vi "Select Excitation Channel.vi"(11 "Sensor List":refnum<class "Sensor List Class.lvclass">) -> (2 "Channel Out":string, 3 "Sensor List Out":refnum<class "Sensor List Class.lvclass">)   [LabVIEW 2013]
uses:
  lib/Data Access Objects/Sensors/Sensor List Class.lvclass
  lib/Data Access Objects/Sensors/Sensor DAO Class.lvclass/Sensor DAO Class.ctl
  <vilib>/regexp/Match Regular Expression.xnode
  lib/Data Access Objects/Sensors/Sensor DAO Class.lvclass
panel:
  in  "Select Excitation Channel":i32[](listbox)
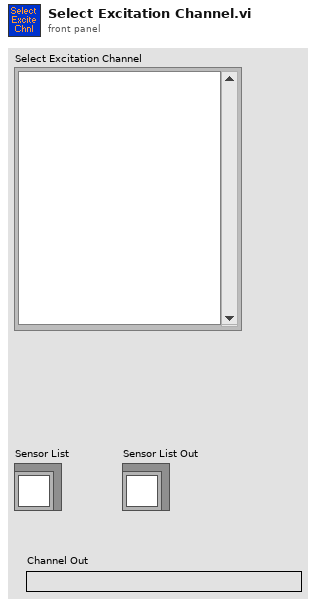
[diagram p1: front panel]
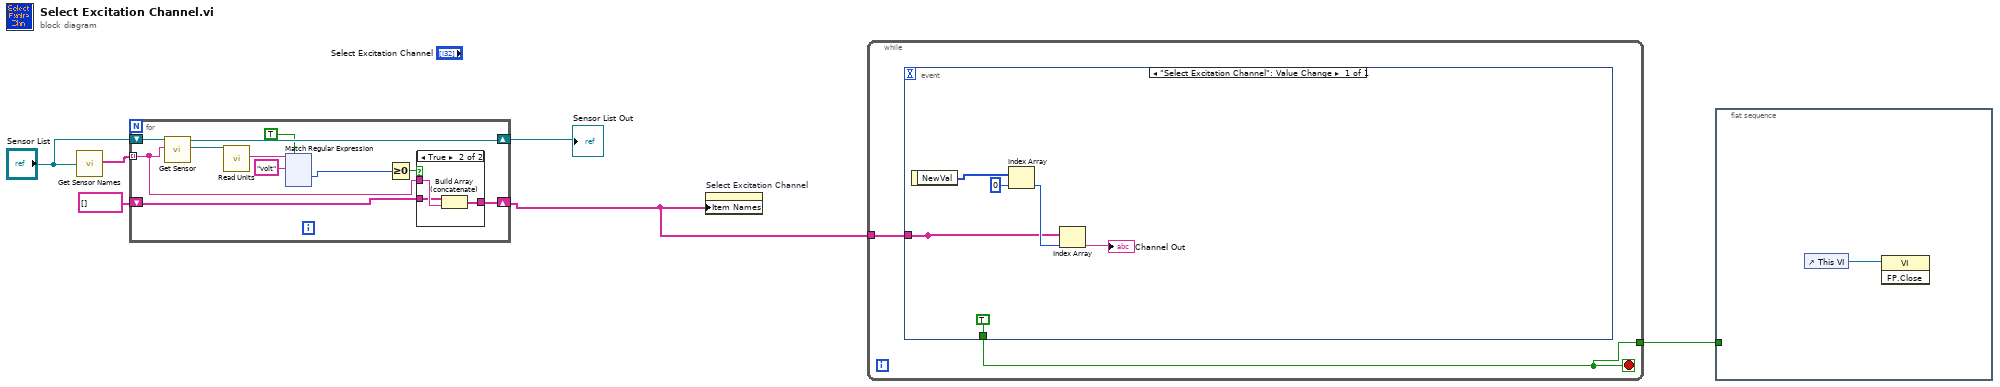
[diagram p0: block diagram]
diagram:
  n1 = call "Get Sensor Names.vi"("Sensor List Class in"="Sensor List") -> ("Names"=w4:string[])  [unwired: 8 in, 2 out]
  n2 = for {
    shift-right: [w17] -> w3
    shift-left: string[] [] -> [w16]
    tunnel: w4 -> [w7] mode=indexing
    shift-right: [w14] -> w1
    shift-left: "Sensor List" -> [w15]
    n3 = call "Get Sensor.vi"("Name"=w7, "Sensor List Class in"=w15) -> ("Sensor DAO Out"=w13:refnum<class "Sensor DAO Class.lvclass">, "Sensor List Class out"=w14:refnum<class "Sensor List Class.lvclass">)  [unwired: 7 in, 1 out]
    n4 = call "Read Units.vi"("Sensor DAO Class in"=w13) -> ("Units"=w12:string)  [unwired: 8 in, 2 out]
    n5 = xnode "Match Regular Expression"("input string"=w12, "regular expression"="volt", "ignore case? (F)"=TRUE) -> ("offset past match"=w10:i32)  [unwired: 3 in, 4 out]
    n6 = Greater Or Equal To 0?(x=w10) -> (x >= 0?=w11:bool)
    n7 = case shown="True" w11 {
      tunnel: w7 -> [_ w135]
      tunnel: [w132 w134] -> w17
      tunnel: w16 -> [w132 w133]
      frame False {
      }
      frame True {
        n8 = Build Array (concatenate)(w133, w135) -> (w134:string[])
      }
    }
  }
  "Sensor List Out" <- w1
  n9 = property on="Select Excitation Channel" class="LstBox (strict)"("Item Names"=w3) -> ()  [unwired: 2 in, 2 out]
  n10 = while {
    tunnel: w3 -> [w137]
    tunnel: [w136] -> w2
    stop <- w136 stop-if-true
    n11 = event shown="[0] \"Select Excitation Channel\": Value Change" {
      selector: _ -> [_]
      dyn-events: _ -> [_]
      timeout: _ -> [_]
      tunnel: [TRUE] -> w136
      tunnel: [w140] -> _
      tunnel: w137 -> [w140]
      event "Select Excitation Channel": Value Change {
        n12 = event-data() -> ("NewVal"=w143:i32[])  [unwired: 1 in]
        n13 = Index Array(array=w143, index=0) -> (element=w141:i32)
        n14 = Index Array(array=w140, index=w141) -> (element=→"Channel Out":string)
      }
    }
  }
  n15 = flat-sequence {
    tunnel: w2 -> [_]
    frame #0 {
      n16 = control-ref of="This VI"() -> (w144:refnum<vi>)
      n17 = invoke class="VI" method="FP.Close"(reference=w144) -> ()  [unwired: 2 in, 3 out]
    }
  }
